vi "Get Sclera Ratio.vi"(8 "Error In":errorcluster, 11 "Image":T1) -> (0 "Error Out":errorcluster, 3 "Sclera Ratio":dbl)   [LabVIEW 2015]
uses:
  <vilib>/vision/Image Controls.llb/IMAQ Image.ctl
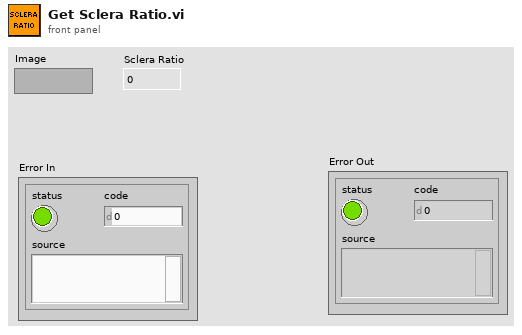
[diagram p1: front panel]
types:
  T1 = typedef "IMAQ Image.ctl" = refnum<image>
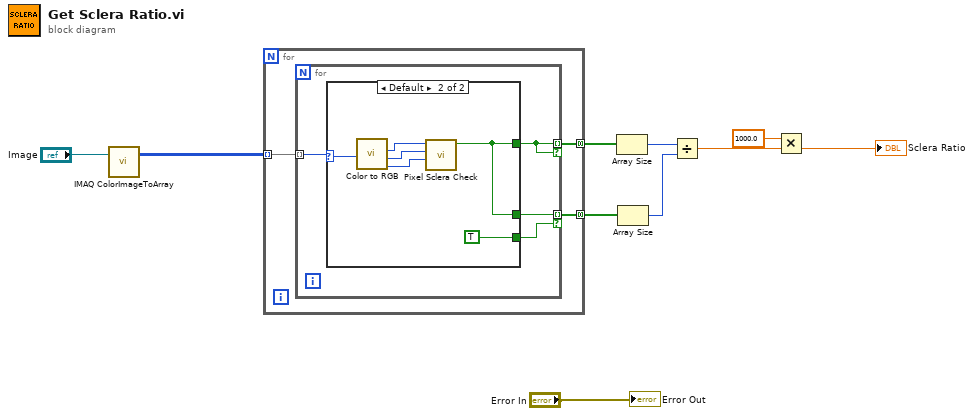
[diagram p0: block diagram]
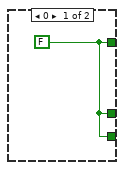
[diagram p2: hidden frame]
diagram:
  n1 = call "IMAQ ColorImageToArray"("Image"="Image") -> ("Image Pixels (U32)"=w8:u32[][])  [unwired: 3 in, 2 out]
  n2 = for {
    tunnel: w8 -> [w13] mode=indexing
    tunnel: [w12] -> w7 mode=concatenating
    tunnel: [w11] -> w9 mode=concatenating
    n3 = for {
      tunnel: w13 -> [w17] mode=indexing
      tunnel: [w14] -> w12 mode=indexing if=w14
      tunnel: [w16] -> w11 mode=indexing if=w15
      n4 = case shown="Default" w17 {
        selector: w17 -> [_ w24]
        tunnel: [w18 w20] -> w14
        tunnel: [w18 w20] -> w16
        tunnel: [w18 TRUE ("RGB Sclera")] -> w15
        frame 0 {
          w18 = FALSE ("RGB Sclera")
        }
        frame Default {
          n5 = call <vilib>:"Color to RGB.vi"("Color"=w24) -> ("R"=w23:u8, "G"=w22:u8, "B"=w21:u8)  [unwired: 1 out]
          n6 = call "Pixel Sclera Check.vi"("Blue"=w21, "Green"=w22, "Red"=w23) -> ("RGB Sclera"=w20:bool)  [unwired: 8 in]
        }
      }
    }
  }
  n7 = Array Size(array=w7) -> (size(s)=w5:i32)
  n8 = Array Size(array=w9) -> (size(s)=w10:i32)
  n9 = Divide(x=w5, y=w10) -> (x/y=w6:dbl)
  n10 = Multiply(x=1000.0, y=w6) -> (x*y=→"Sclera Ratio":dbl)
  "Error Out" <- "Error In"
